vi "AlliGator Wait for Test Result [no Error].vi"(8 "error in (no error)":errorcluster, 9 "Time out (10 s)":dbl=10.0) -> (0 "error out":errorcluster)   [LabVIEW 2021]
uses:
  <vilib>/Utility/error.llb/Error Cluster From Error Code.vi
  <vilib>/ErrorRing/Error Ring.xnode
  Time/Time.lvlib
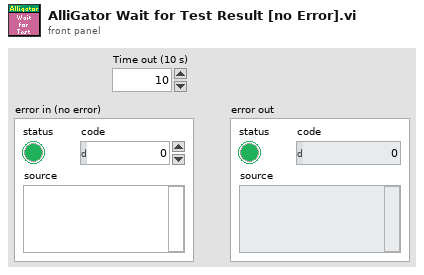
[diagram p1: front panel]
types:
  T1 = enum16{"Store Test Name", "Store Test Result", "Read Test Result"}
  T2 = typedef "AlliGator Test Data.ctl" = cluster{"Test String":string, "error":errorcluster, "Status":bool}
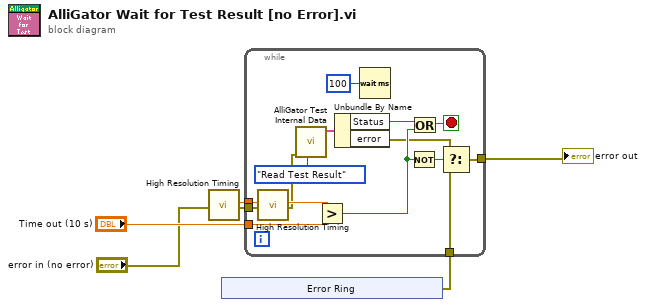
[diagram p0: block diagram]
diagram:
  n1 = call "High Resolution Timing.vi"("Error In"="error in (no error)") -> ("elapsed (relative) seconds"=w3:dbl, "Error Out"=w2:errorcluster)  [unwired: 16 in, 1 out]
  n2 = xnode "Error Ring"() -> ("error out"=w6:errorcluster)
  n3 = while {
    tunnel: [w12] -> w1
    tunnel: w3 -> [w18]
    tunnel: "Time out (10 s)" -> [w16]
    tunnel: w6 -> [w9]
    tunnel: w2 -> [w8]
    stop <- w15 stop-if-true
    n4 = call "High Resolution Timing.vi"("relative seconds (NaN)"=w18, "Error In"=w8) -> ("elapsed (relative) seconds"=w17:dbl, "Error Out"=w7:errorcluster)  [unwired: 15 in, 1 out]
    n5 = call "AlliGator Test Internal Data.vi"("Test State"=T1."Read Test Result", "Error In"=w7) -> ("AlliGator Test Data"=w19:T2)  [unwired: 8 in, 1 out]
    n6 = Greater?(x=w17, y=w16) -> (0:w13:bool)
    n7 = Unbundle By Name(w19) -> ("Status"=w14:bool, "error"=w11:errorcluster)
    n8 = Wait (ms)(milliseconds to wait=u32 100) -> ()  [unwired: 1 out]
    n9 = Not(x=w13) -> (.not. x?=w10:bool)
    n10 = Or(x=w14, y=w13) -> (x .or. y?=w15:bool)
    n11 = Select(t=w11, s=w10, f=w9) -> (s? t:f=w12:errorcluster)
  }
  "error out" <- w1
